vi "GetLiveVolume.vi"(8 "error in":errorcluster, 10 "VolumeQueueIN":refnum<queue>) -> (0 "error out 2":errorcluster, 1 "VolumeOut":u16[][](array[numeric]))   [LabVIEW 2015]
uses:
  NIDAQControls/NIDAQGlobals.vi
  AcquisitionGlobals.vi
panel:
  out "Numeric":i32
  out "size(s)":i32[](array[numeric])
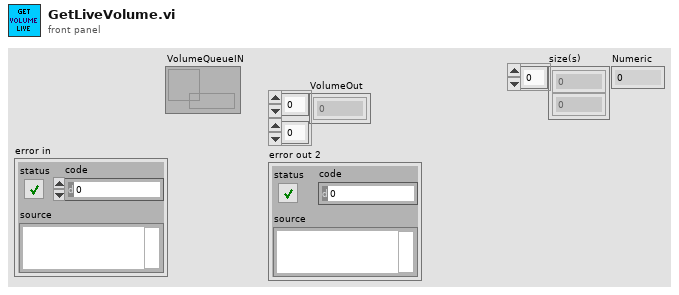
[diagram p1: front panel]
types:
  T1 = enum16{"Create", "Lossy Enqueue", "Enqueue", "Dequeue", "Destroy"}
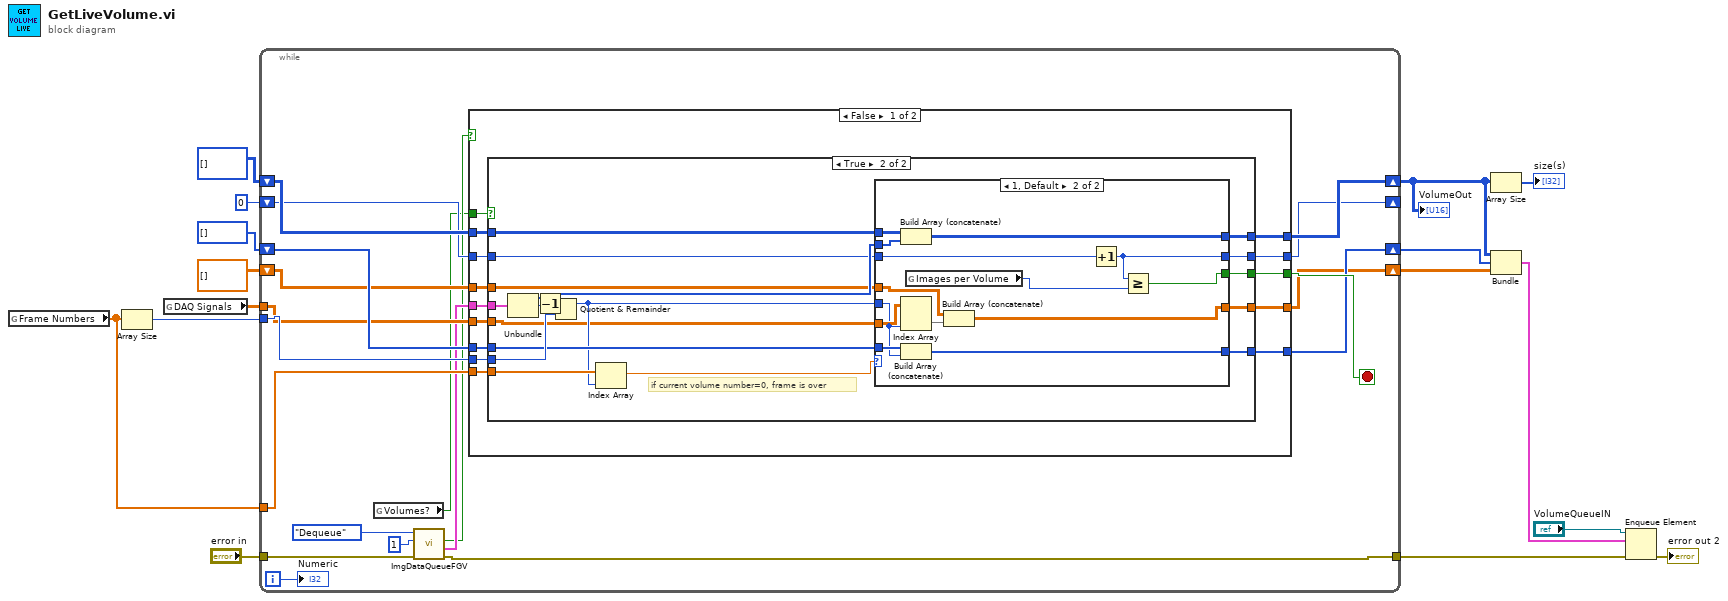
[diagram p0: block diagram]
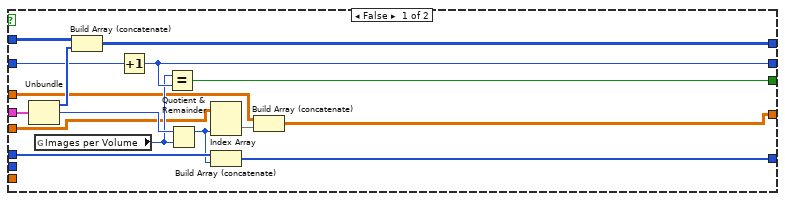
[diagram p2: hidden frame]
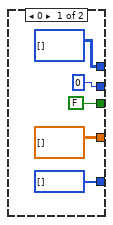
[diagram p3: hidden frame]
diagram:
  n1 = global read "NIDAQGlobals.vi" "Frame Numbers"() -> (w16:dbl[])
  n2 = Array Size(array=w16) -> (size(s)=w15:i32)
  n3 = global read "NIDAQGlobals.vi" "DAQ Signals"() -> (w7:dbl[][])
  n4 = while {
    tunnel: "error in" -> [w20]
    tunnel: w16 -> [w36]
    tunnel: w15 -> [w35]
    shift-right: [w34] -> w2
    shift-left: u16[][] [] -> [w33]
    shift-right: [w30] -> _
    shift-left: u16 0 ("x") -> [w31]
    tunnel: [w19] -> w11
    shift-right: [w28] -> w8
    shift-left: i32[] [] -> [w29]
    tunnel: w7 -> [w27]
    shift-right: [w26] -> w6
    shift-left: dbl[][] [] -> [w25]
    i -> [w17]
    stop <- w32 stop-if-true
    n5 = global read "AcquisitionGlobals.vi" "Volumes?"() -> (w18:bool)
    n6 = call "ImgDataQueueFGV.vi"("error out"=w20, "timeout in ms (-1)"=1, "Action"=T1."Dequeue") -> ("error out 2"=w19:errorcluster, "Data Out"=w23:cluster{u16[], i32, i64}, "timed out?"=w21:bool)  [unwired: 6 in]
    n7 = case shown="False" w21 {
      tunnel: w36 -> [w50 _]
      tunnel: w35 -> [w49 _]
      tunnel: [w48 w107] -> w34
      tunnel: w33 -> [w47 w107]
      tunnel: [w46 _] -> w32
      tunnel: w31 -> [w45 w104]
      tunnel: [w44 w104] -> w30
      tunnel: w29 -> [w43 w106]
      tunnel: [w42 w106] -> w28
      tunnel: w27 -> [w41 _]
      tunnel: [w40 w105] -> w26
      tunnel: w25 -> [w39 w105]
      tunnel: w23 -> [w38 _]
      tunnel: w18 -> [w37 _]
      frame False {
        n8 = case shown="True" w37 {
          tunnel: w50 -> [_ w84]
          tunnel: w49 -> [_ w83]
          tunnel: [w64 w81] -> w48
          tunnel: w47 -> [w58 w80]
          tunnel: [w61 w79] -> w46
          tunnel: w45 -> [w60 w78]
          tunnel: [w59 w77] -> w44
          tunnel: w43 -> [w62 w75]
          tunnel: [w63 w73] -> w42
          tunnel: w41 -> [w55 w72]
          tunnel: [w52 w71] -> w40
          tunnel: w39 -> [w51 w69]
          tunnel: w38 -> [w66 w70]
          frame False {
            n9 = Unbundle(w66) -> (w65:u16[], w57:i32)  [unwired: 1 out]
            n10 = global read "NIDAQGlobals.vi" "Images per Volume"() -> (w56:u16)
            n11 = Build Array (concatenate)(w58, w65) -> (w64:u16[][])
            n12 = Increment(x=w60) -> (x+1=w59:u16)
            n13 = Equal?(x=w56, y=w59) -> (x = y?=w61:bool)
            n14 = Quotient & Remainder(x=w57, y=w56) -> (x-y*floor(x/y)=w54:i32)  [unwired: 1 out]
            n15 = Index Array(array=w55, index (col)=w54) -> (element=w53:dbl[])  [unwired: 1 in]
            n16 = Build Array (concatenate)(w62, w54) -> (w63:i32[])
            n17 = Build Array (concatenate)(w51, w53) -> (w52:dbl[][])
          }
          frame True {
            # "if current volume number=0, frame is over"
            n18 = Unbundle(w70) -> (w82:u16[], w76:i32)  [unwired: 1 out]
            n19 = Decrement(x=w76) -> (x-1=w67:i32)
            n20 = Quotient & Remainder(x=w67, y=w83) -> (x-y*floor(x/y)=w74:i32)  [unwired: 1 out]
            n21 = Index Array(array=w84, index=w74) -> (element=w68:dbl)
            n22 = case shown="1, Default" w68 {
              tunnel: w82 -> [_ w103]
              tunnel: [u16[][] [] w102] -> w81
              tunnel: w80 -> [_ w101]
              tunnel: [FALSE w99] -> w79
              tunnel: w78 -> [_ w98]
              tunnel: [u16 0 ("x") w97] -> w77
              tunnel: w74 -> [_ w93]
              tunnel: [i32[] [] w96] -> w73
              tunnel: w75 -> [_ w95]
              tunnel: w72 -> [_ w94]
              tunnel: [dbl[][] [] w91] -> w71
              tunnel: w69 -> [_ w90]
              frame 0 {
              }
              frame 1, Default {
                n23 = Build Array (concatenate)(w101, w103) -> (w102:u16[][])
                n24 = Index Array(array=w94, index (col)=w93) -> (element=w92:dbl[])  [unwired: 1 in]
                n25 = Build Array (concatenate)(w95, w93) -> (w96:i32[])
                n26 = global read "NIDAQGlobals.vi" "Images per Volume"() -> (w100:u16)
                n27 = Build Array (concatenate)(w90, w92) -> (w91:dbl[][])
                n28 = Increment(x=w98) -> (x+1=w97:u16)
                n29 = Greater Or Equal?(x=w97, y=w100) -> (x >= y?=w99:bool)
              }
            }
          }
        }
      }
      frame True {
      }
    }
    "Numeric" <- w17
  }
  "VolumeOut" <- w2
  n30 = Array Size(array=w2) -> (size(s)=→"size(s)":i32[])
  n31 = Bundle(w2, w8, w6) -> (w3:cluster{u16[][], i32[], dbl[][]})  [unwired: 1 in]
  n32 = Enqueue Element(queue="VolumeQueueIN", element=w3, error in (no error)=w11) -> (error out=→"error out 2":errorcluster)  [unwired: 1 in, 2 out]
